vi "point_to_time_4.vi"() -> ()   [LabVIEW 2016]
panel:
  out "dt (us)":dbl
  out "Pulse Width (us)":dbl
  in  "number of points":i32
  out "time (us)":dbl
  in  "DAC frequency(MHz)":dbl
  in  "point location":i32
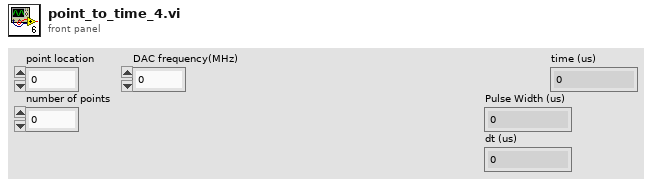
[diagram p1: front panel]
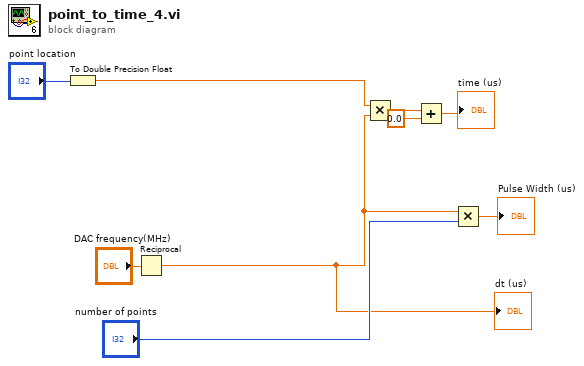
[diagram p0: block diagram]
diagram:
  n1 = To Double Precision Float(number="point location") -> (double precision float=w4:dbl)
  n2 = Reciprocal(x="DAC frequency(MHz)") -> (1/x=w6:dbl)
  "dt (us)" <- w6
  n3 = Multiply(x=w4, y=w6) -> (x*y=w2:dbl)
  n4 = Add(x=w2, y=0.0) -> (x+y=→"time (us)":dbl)
  n5 = Multiply(x=w6, y="number of points") -> (x*y=→"Pulse Width (us)":dbl)
